vi "BrokenVI.vi"(8 "Numeric":dbl=4.0) -> (0 "Numeric 2":dbl)   [LabVIEW 2023]
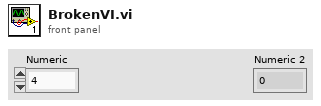
[diagram p1: front panel]
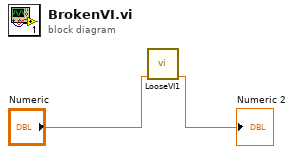
[diagram p0: block diagram]
diagram:
  n1 = call "LooseVI1.vi"("Numeric"="Numeric") -> ("Numeric 2"=→"Numeric 2":dbl)  [unwired: 10 in]
